vi "Launch Subordinate.vi"(6 "PanelIndex":i32, 7 "Identifier":string, 8 "error in (no error)":errorcluster, 9 "Panel":refnum<class "Panel.lvclass">, 10 "Nested Panel Actor":refnum<class "Panel Actor.lvclass">, 11 "Managed Actor in":refnum<class "Managed Actor.lvclass">) -> (0 "error out":errorcluster, 2 "Subordinate":T1, 3 "Managed Actor out":refnum<class "Managed Actor.lvclass">)   [LabVIEW 2023, in "Engine.lvlib" / "Managed Actor.lvlib" / "Managed Actor.lvclass"]
doc: "<b>Launch Subordinate</b> Calls the Panel Manager method <b>Launch Nested PanelActor</b> which launches a new nested Panel Actor with the specified panel type.\n\nIt returns a subordinate record which must be inserted into the managed actor's map for administration."
uses:
  Library/Managed Actor.lvclass
  builds/Framework/Panel Manager.lvlibp/Library/Panel Actor.lvclass
  builds/Framework/Panel Manager.lvlibp/Panel/Panel/Panel.lvclass
  Custom Controls/Subordinate.ctl
  builds/Framework/Actor Framework.lvlibp/1abvi3w/vi.lib/ActorFramework/Message Enqueuer/Message Enqueuer.lvclass
  builds/Framework/Actor Framework.lvlibp/1abvi3w/vi.lib/ActorFramework/Actor/Write Actor Label.vi
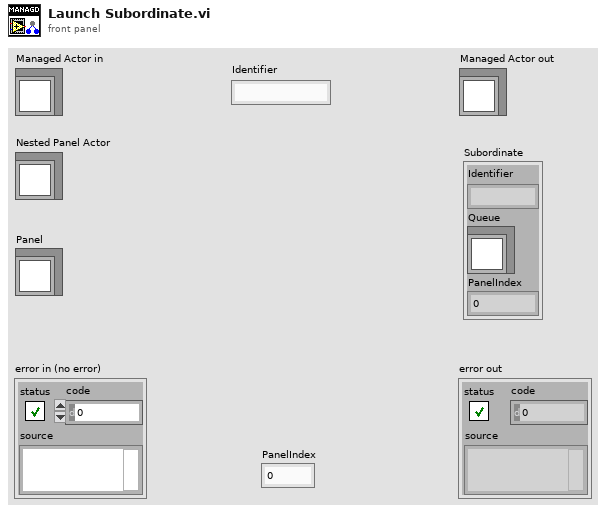
[diagram p1: front panel]
types:
  T1 = typedef "Engine.lvlib/Managed Actor.lvlib/Managed Actor.lvclass/Subordinate.ctl" = cluster{"Identifier":string, "Queue":refnum<class "Message Enqueuer.lvclass">, "PanelIndex":i32}
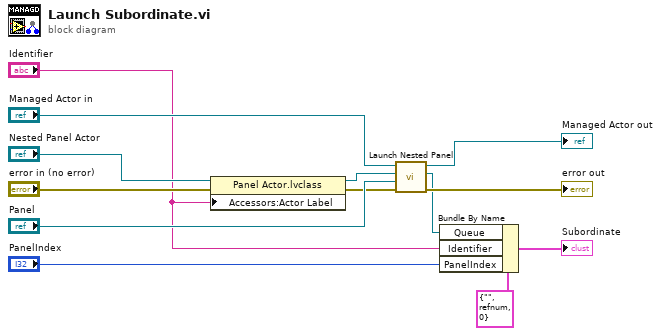
[diagram p0: block diagram]
diagram:
  n1 = property class="Panel Actor.lvclass"(reference="Nested Panel Actor", error in="error in (no error)", "Accessors:Actor Label"="Identifier") -> (reference out=w9:refnum<class "Panel Actor.lvclass">, error out=w8:errorcluster)
  n2 = call "Launch Nested Panel.vi"("error in (no error)"=w8, "Panel"="Panel", "Nested Panel Actor"=w9, "Panel Actor in"="Managed Actor in") -> ("error out"=→"error out":errorcluster, "Nested Actor's Enqueuer"=w4:refnum<class "Message Enqueuer.lvclass">, "Panel Actor out"=→"Managed Actor out":refnum<class "Managed Actor.lvclass">)  [unwired: 4 in, 1 out]
  n3 = Bundle By Name(cluster=T1 {"Identifier"="", "Queue"=refnum, "PanelIndex"=0} ("Subordinate"), "Queue"=w4, "Identifier"="Identifier", "PanelIndex"="PanelIndex") -> (→"Subordinate":T1)
